vi "Set Tag.vi"(8 "Error In":errorcluster, 10 "Tag":string, 11 "Animation In":refnum<class "Animation.lvclass">) -> (0 "Error Out":errorcluster, 3 "Animation Out":refnum<class "Animation.lvclass">)   [LabVIEW 2021, in "Animation.lvclass"]
uses:
  Animation.lvclass
  Animation.lvclass/Animation.ctl
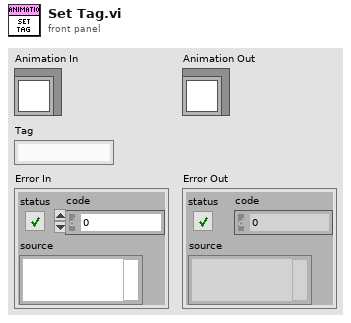
[diagram p1: front panel]
types:
  T1 = typedef "Animation.lvclass/Data.ctl" = cluster{"Tag":string}
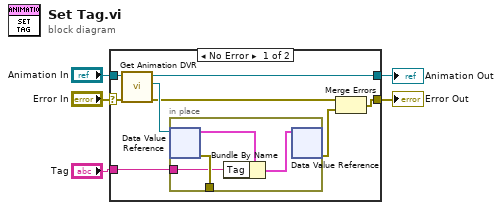
[diagram p0: block diagram]
diagram:
  n1 = case shown="No Error" "Error In" {
    selector: "Error In" -> [w9 w18]
    tunnel: [w12 w18] -> w4
    tunnel: [w7 w19] -> w2
    tunnel: "Animation In" -> [w10 w19]
    tunnel: "Tag" -> [w11 _]
    frame No Error {
      n2 = call "Get Animation DVR.vi"("Error In"=w9, "Animation In"=w10) -> ("Error Out"=w6:errorcluster, "DVR"=w8:refnum<data-value>, "Animation Out"=w7:refnum<class "Animation.lvclass">)  [unwired: 7 in]
      n3 = in-place {
        in-place-border: [w17] -> _
        in-place-border: w11 -> [w14]
        n4 = in-place-dvr #1(w8) -> (w16:T1, w17:errorcluster)
        n5 = Bundle By Name(cluster=w16, "Tag"=w14) -> (w15:T1)
        n6 = in-place-dvr #1(w15) -> (w13:errorcluster)  [unwired: 1 out]
      }
      n7 = Merge Errors(w6, w13) -> (w12:errorcluster)
    }
    frame Error {
    }
  }
  "Animation Out" <- w2
  "Error Out" <- w4
